vi "PBI_MFA_Interface_DriveDisable.vi"() -> (2 "DriveEnable":bool, 3 "status":bool)   [LabVIEW 2011]
panel:
  out "error DriveEnableOut":errorcluster
  out "error DriveEnableIn":errorcluster
  out "AAABuild":i32
  in  "MintController":refnum<k7>(container)
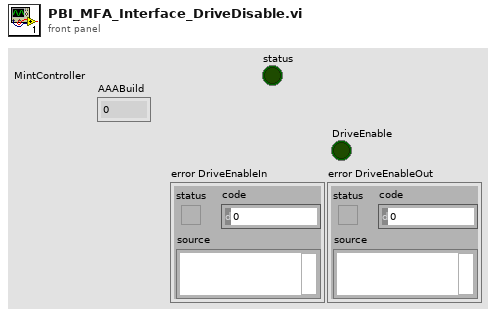
[diagram p1: front panel]
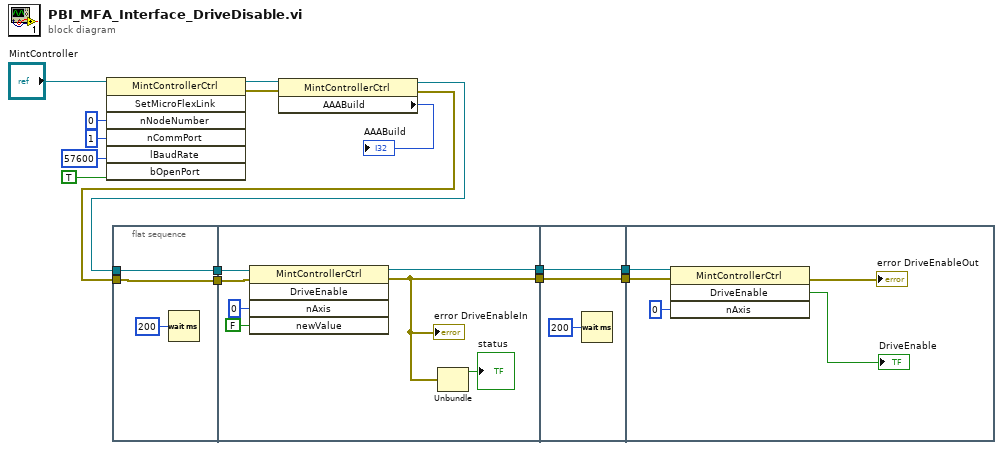
[diagram p0: block diagram]
diagram:
  n1 = invoke class="MintControllerCtrl" method="SetMicroFlexLink"(reference="MintController", "nNodeNumber"=i16 0, "nCommPort"=i16 1, "lBaudRate"=57600, "bOpenPort"=TRUE) -> (reference out=w16:refnum<k7>, error out=w10:errorcluster)  [unwired: 2 in, 5 out]
  n2 = flat-sequence {
    tunnel: w4 -> [w18]
    tunnel: w3 -> [w17]
    tunnel: [w18] -> w2
    tunnel: [w17] -> w1
    tunnel: [w21] -> w7
    tunnel: [w24] -> w5
    tunnel: w2 -> [w23]
    tunnel: w1 -> [w22]
    tunnel: [w28] -> w8
    tunnel: w7 -> [w28]
    tunnel: [w27] -> w6
    tunnel: w5 -> [w27]
    tunnel: w8 -> [w33]
    tunnel: w6 -> [w34]
    frame #0 {
      n3 = Wait (ms)(milliseconds to wait=u32 200) -> ()  [unwired: 1 out]
    }
    frame #1 {
      n4 = invoke class="MintControllerCtrl" method="DriveEnable"(reference=w23, error in=w22, "nAxis"=i16 0, "newValue"=FALSE) -> (reference out=w24:refnum<k7>, error out=w21:errorcluster)  [unwired: 1 in, 3 out]
      "error DriveEnableIn" <- w21
      n5 = Unbundle(w21) -> ("status"=→"status":bool)  [unwired: 2 out]
    }
    frame #2 {
      n6 = Wait (ms)(milliseconds to wait=u32 200) -> ()  [unwired: 1 out]
    }
    frame #3 {
      n7 = invoke class="MintControllerCtrl" method="DriveEnable"(reference=w34, error in=w33, "nAxis"=i16 0) -> (error out=→"error DriveEnableOut":errorcluster, "DriveEnable"=→"DriveEnable":bool)  [unwired: 1 in, 2 out]
    }
  }
  n8 = property class="MintControllerCtrl"(reference=w16, error in=w10) -> (reference out=w4:refnum<k7>, error out=w3:errorcluster, "AAABuild"=→"AAABuild":i32)
